vi "CSM - Config MassData Parameter Cache Size.vi"(9 "Error in":errorcluster caption="Error in (no error)", 10 "Size (50M)":i32=50000000 format="%.0p") -> (1 "Error out":errorcluster)   [LabVIEW 2017, in "CSM MassData Parameter Support.lvlib"]
doc: "Configures the Massdata background cache size. The default value is 50 MB.\n\nIt is recommended to configure an appropriate cache size that is not too large to avoid wasting memory and not too small to prevent frequent overwrites. You can use the provided debugging tools to monitor cache usage and determine the optimal configuration.\n\n> [!WARNING]\n> DO NOT adjust the cache size while the application is running. Adjusting the cache size will reallocate memory, potentially leading to data loss.\n> It is recommended to configure the cache size before application startup to ensure it meets the application's requirements.\n\n\n> [!NOTE] <b>CSM Massdata Argument Support</b>\n>\n> CSM Massdata argument support provides an efficient argument passing mechanism for transferring large amounts of data within CSM. By using a memory-efficient reference mechanism instead of direct data transfer, CSM Massdata improves the efficiency and performance of argument passing.\n> - The argument type defined by CSM Massdata is `<MassData>`, which can be obtained using the CSM - Argument Type VI.\n> - Data transmission of CSM Massdata is completely lossless. However, it is not suitable for storing data that requires indefinite persistence.\n>\n> <b>Note</b>: CSM Massdata internally uses a circular buffer mechanism. All CSM modules within the same application share the same Massdata buffer space. When the buffer is full, new data will overwrite old data starting from the beginning. Therefore, you need to set a reasonable buffer size to ensure that data is not overwritten before use, avoiding data loss.\n\n\n-- <b>Controls</b> --\n- <b>Size (50M)</b>: Cache size in bytes. The default is 50 MB."
uses:
  CSM MassData Parameter Support.lvlib
  _support/Operation-FGV-MassData.ctl
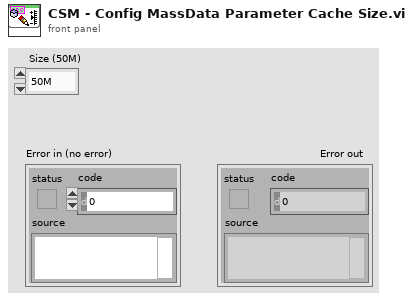
[diagram p1: front panel]
types:
  T1 = typedef "CSM MassData Parameter Support.lvlib/Operation-FGV-MassData.ctl" = enum16{"Initialize", "Read", "Write", "Status", "Release"}
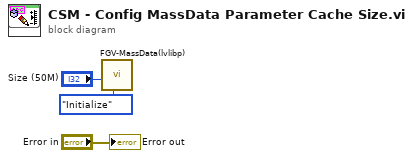
[diagram p0: block diagram]
diagram:
  n1 = call "FGV-MassData(lvlibp).vi"("Operation"=Operation-FGV-MassData."Initialize", "size"="Size (50M)") -> ()  [unwired: 6 in, 4 out]
  "Error out" <- "Error in"
